vi "filter array by pattern.vi"(10 "Array In":string[](array[string]), 11 "Pattern In":string) -> (3 "Filtered Array":i32[](array[numeric]))   [LabVIEW 2020]
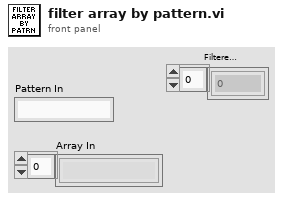
[diagram p1: front panel]
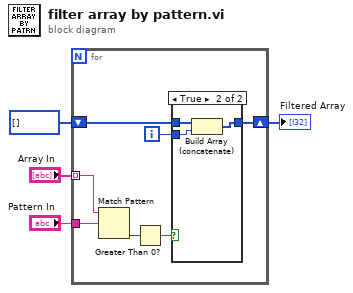
[diagram p0: block diagram]
diagram:
  n1 = for {
    tunnel: "Array In" -> [w11] mode=indexing
    tunnel: "Pattern In" -> [w10]
    shift-right: [w5] -> w1
    shift-left: i32[] [] -> [w7]
    i -> [w6]
    n2 = Match Pattern(string=w11, regular expression=w10) -> (offset past match=w9:i32)  [unwired: 1 in, 3 out]
    n3 = Greater Than 0?(x=w9) -> (x > 0?=w8:bool)
    n4 = case shown="True" w8 {
      tunnel: w7 -> [w12 w15]
      tunnel: w6 -> [_ w14]
      tunnel: [w12 w13] -> w5
      frame False {
      }
      frame True {
        n5 = Build Array (concatenate)(w15, w14) -> (w13:i32[])
      }
    }
  }
  "Filtered Array" <- w1
